vi "3-9.vi"() -> ()   [LabVIEW 2014]
panel:
  in  "Max Wind Speed":dbl
  in  "Current Wind Speed":dbl
  out "?":string
  out "Warning?":bool
  in  "Min Temp.":dbl
  in  "Max Temp.":dbl
  in  "Current Temp.":dbl
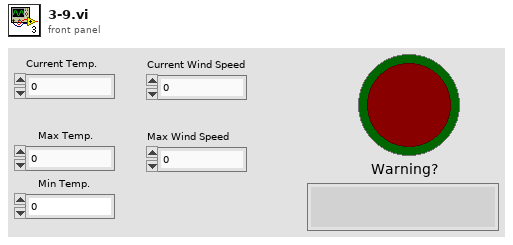
[diagram p1: front panel]
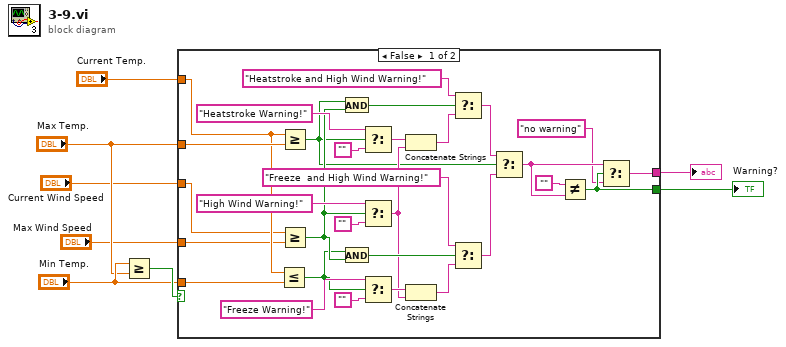
[diagram p0: block diagram]
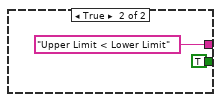
[diagram p2: hidden frame]
diagram:
  n1 = Greater Or Equal?(x="Min Temp.", y="Max Temp.") -> (x >= y?=w8:bool)
  n2 = case shown="False" w8 {
    tunnel: [w11 "Upper Limit < Lower Limit"] -> w7
    tunnel: [w12 TRUE] -> w6
    tunnel: "Current Temp." -> [w36 _]
    tunnel: "Min Temp." -> [w35 _]
    tunnel: "Max Temp." -> [w38 _]
    tunnel: "Current Wind Speed" -> [w33 _]
    tunnel: "Max Wind Speed" -> [w32 _]
    frame False {
      n3 = Less Or Equal?(x=w36, y=w35) -> (x <= y?=w29:bool)
      n4 = Greater Or Equal?(x=w36, y=w38) -> (x >= y?=w16:bool)
      n5 = Greater Or Equal?(x=w33, y=w32) -> (x >= y?=w30:bool)
      n6 = And(x=w16, y=w30) -> (x .and. y?=w28:bool)
      n7 = And(x=w29, y=w30) -> (x .and. y?=w21:bool)
      n8 = Select(t="Heatstroke Warning!", s=w16, f="") -> (s? t:f=w22:string)
      n9 = Select(t="High Wind Warning!", s=w30, f="") -> (s? t:f=w18:string)
      n10 = Select(t="Freeze Warning!", s=w29, f="") -> (s? t:f=w19:string)
      n11 = Concatenate Strings(w22, w18) -> (w23:string)
      n12 = Concatenate Strings(w19, w18) -> (w17:string)
      n13 = Select(t="Heatstroke and High Wind Warning!", s=w28, f=w23) -> (s? t:f=w15:string)
      n14 = Select(t="Freeze  and High Wind Warning!", s=w21, f=w17) -> (s? t:f=w14:string)
      n15 = Select(t=w15, s=w16, f=w14) -> (s? t:f=w10:string)
      n16 = Not Equal?(x="", y=w10) -> (x != y?=w12:bool)
      n17 = Select(t=w10, s=w12, f="no warning") -> (s? t:f=w11:string)
    }
    frame True {
    }
  }
  "Warning?" <- w6
  "?" <- w7
